vi "ObjDet_Read_Dataset.vi"(0 "Image Path(Train)":path, 1 "Validation Portion":sgl, 2 "Rndomize":bool=TRUE, 5 "Anno Path(Train)":path, 7 "Image Path(Test)":path, 9 "Anno Path(Test)":path, 11 "error in (no error)":errorcluster, 12 "Img Height":i32=128, 13 "Img Width":i32=128, 14 "Img Type":enum16{"Grayscale", "RGB"}(ring)) -> (4 "Dataset":T1={"Train"={"Inputs Ref."=variant(refnum<data-value> refnum), "Dataset_Size"=0, "Dims_In"={"C"=0, "H"=0, "W"=0}, "Outputs Refs"=refnum, "No of Classes "=0, "Labels"=["large", "small"], "File Paths"=[]}, "Validation"={"Inputs Ref."=variant(refnum<data-value> refnum), "Dataset_Size"=0, "Dims_In"={"C"=0, "H"=0, "W"=0}, "Outputs Refs"=refnum, "No of Classes "=0, "Labels"=["large", "small"], "File Paths"=[]}, "Test"={"Inputs Ref."=variant(refnum<data-value> refnum), "Dataset_Size"=0, "Dims_In"={"C"=0, "H"=0, "W"=0}, "Outputs Refs"=refnum, "No of Classes "=0, "Labels"=["large", "small"], "File Paths"=[]}}, 6 "Anchors":dbl[][](array[numeric]), 8 "Total annotations":i32, 15 "error out":errorcluster)   [LabVIEW 2020]
uses:
  <vilib>/Ngene/Deep Learning Toolkit/Toolkit/NN_Data/API/DataSet/DataSet_Types/NN_DataSets_All(In3D_OutBBox).ctl
  <vilib>/Ngene/Deep Learning Toolkit/Toolkit/NN_Data/API/DataSet/DataSet_Types/NN_DataSet(In3D_OutBBox).ctl
  <vilib>/Ngene/Deep Learning Toolkit/Toolkit/NN_Data/API/NN_Dims(C,H,W).ctl
  <vilib>/Ngene/Deep Learning Toolkit/Toolkit/NN_Data/Controls/DataRef_Types/1D/NN_Data_ref(1D_BBox).ctl
  <vilib>/Ngene/Deep Learning Toolkit/Toolkit/NN_Data/API/Data/Detection_Types/NN_Image_Annotations.ctl
  <vilib>/Ngene/Deep Learning Toolkit/Toolkit/NN_Data/API/Data/Detection_Types/NN_BBox_Annotation.ctl
  <vilib>/Ngene/Deep Learning Toolkit/Toolkit/NN_Data/API/Data/Detection_Types/NN_BBox.ctl
  <vilib>/Analysis/1siggen.llb/Riffle Array (I32).vi
  <vilib>/Ngene/Deep Learning Toolkit/Toolkit/Deep_Learning_Toolkit_by_Ngene.lvlib
  <vilib>/Analysis/NI_AALBase.lvlib
panel:
  in  "seed":i32=-1
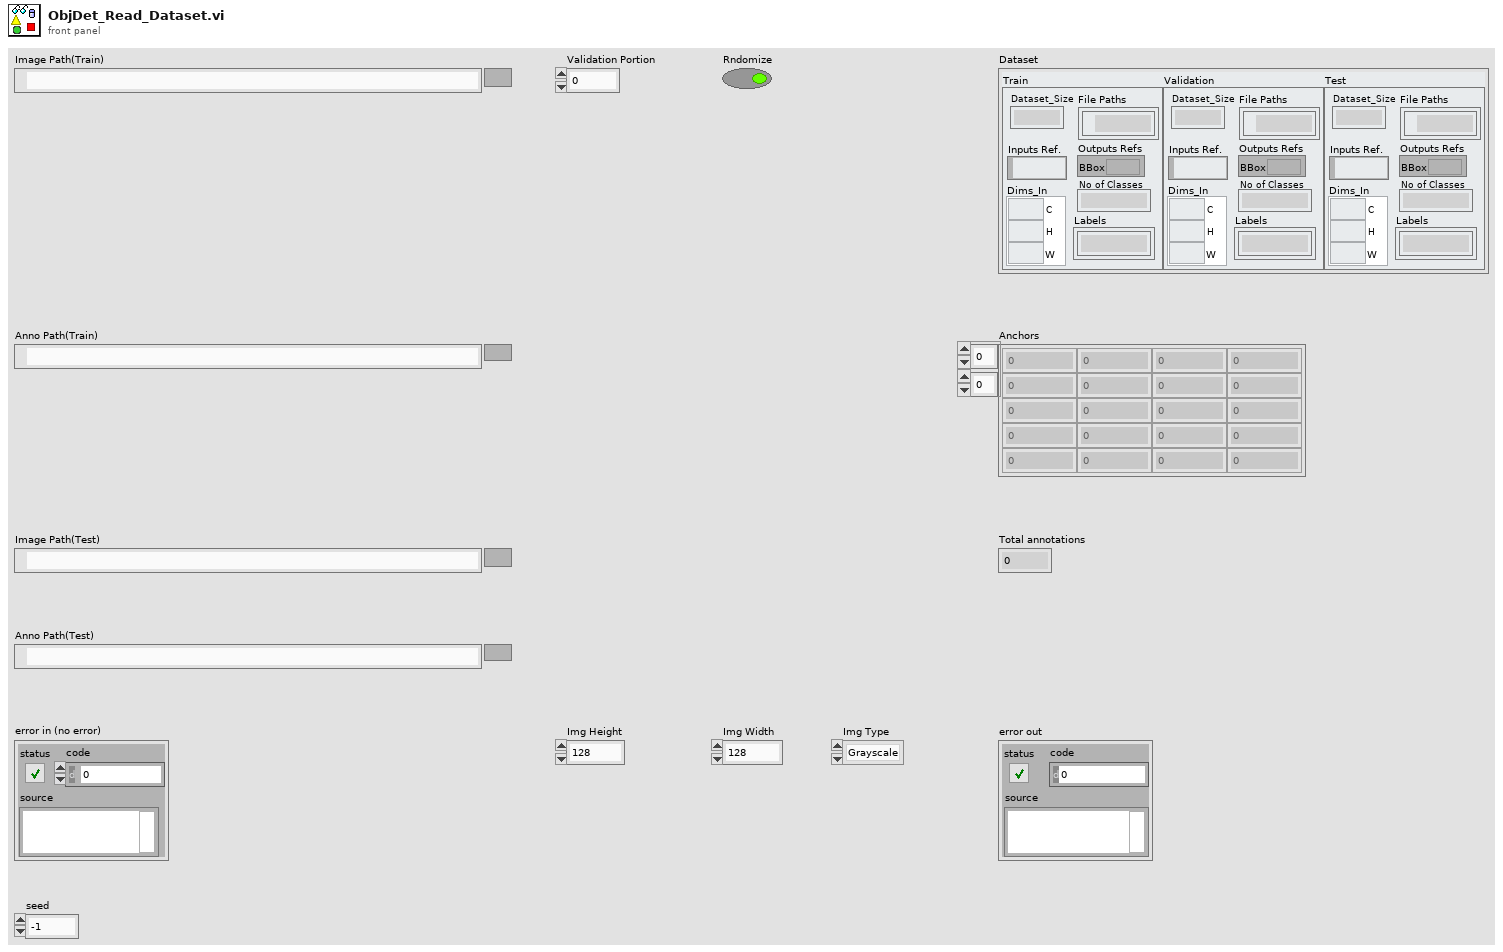
[diagram p1: front panel]
types:
  T1 = typedef "Deep_Learning_Toolkit_by_Ngene.lvlib/NN_DataSets_All(In3D_OutBBox).ctl" = cluster{"Train":T2, "Validation":T2, "Test":T2}
  T2 = typedef "Deep_Learning_Toolkit_by_Ngene.lvlib/NN_DataSet(In3D_OutBBox).ctl" = cluster{"Inputs Ref.":variant, "Dataset_Size":i32, "Dims_In":T3, "Outputs Refs":T4, "No of Classes ":i32, "Labels":string[], "File Paths":path[]}
  T3 = typedef "Deep_Learning_Toolkit_by_Ngene.lvlib/NN_Dims(C,H,W).ctl" = cluster{"C":i32, "H":i32, "W":i32}
  T4 = typedef "Deep_Learning_Toolkit_by_Ngene.lvlib/NN_Data_ref(1D_BBox).ctl" = refnum<data-value>
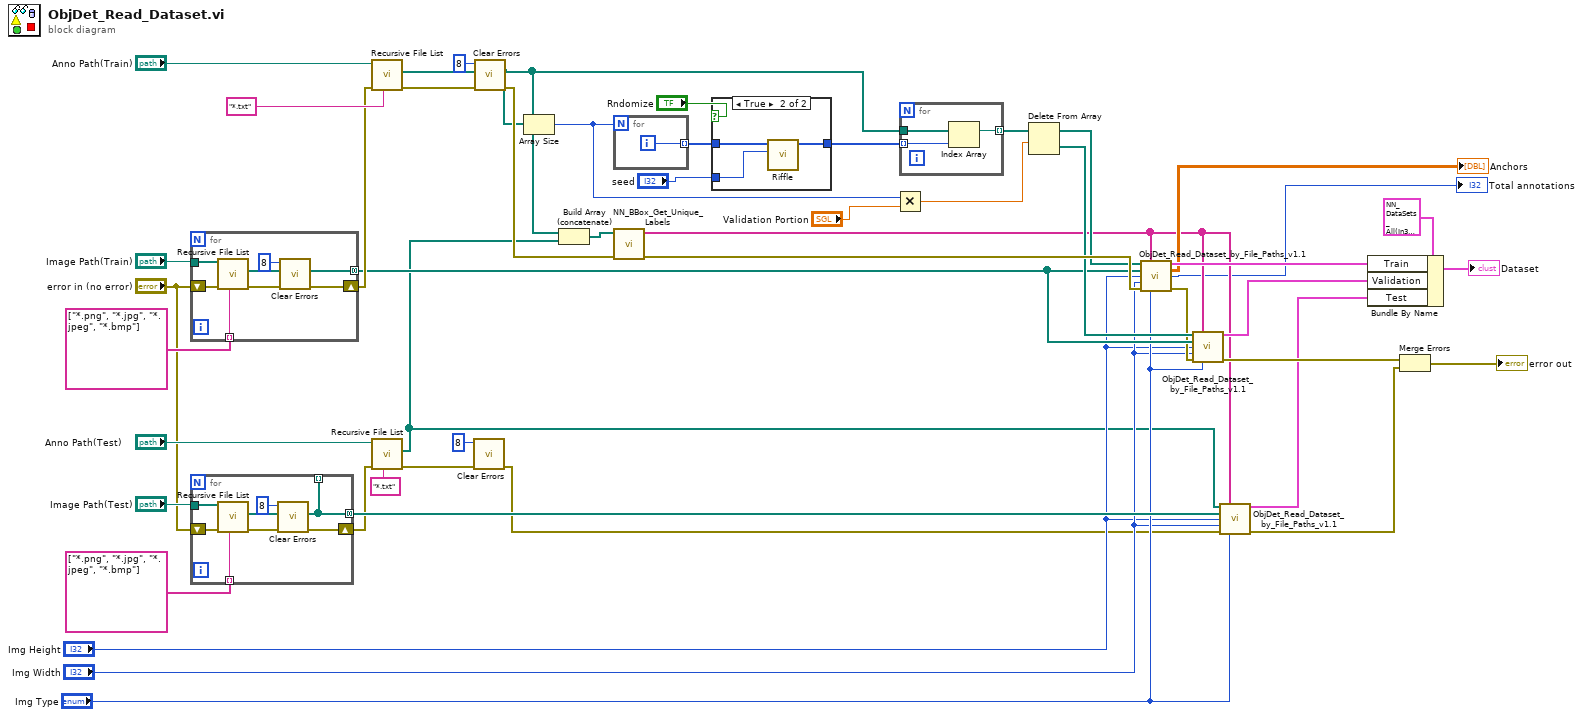
[diagram p0: block diagram]
diagram:
  n1 = for {
    tunnel: "Image Path(Train)" -> [w55]
    tunnel: string[] ["*.png", "*.jpg", "*.jpeg", "*.bmp"] ("pattern") -> [w54] mode=indexing
    tunnel: [w49] -> w31 mode=concatenating
    shift-right: [w51] -> w46
    shift-left: "error in (no error)" -> [w53]
    n2 = call <vilib>:"Recursive File List.vi"("pattern"=w54, "error in (no error)"=w53, "Folder Path"=w55) -> ("error out"=w52:errorcluster, "All Files in Dir"=w49:path[])  [unwired: 4 in, 3 out]
    n3 = call <vilib>:"Clear Errors.vi"("error in (no error)"=w52, "specific error code to clear (0: all)"=8) -> ("error out"=w51:errorcluster)  [unwired: 4 in, 1 out]
  }
  n4 = for {
    tunnel: "Image Path(Test)" -> [w62]
    tunnel: string[] ["*.png", "*.jpg", "*.jpeg", "*.bmp"] ("pattern") -> [w61] mode=indexing
    tunnel: [w56] -> w26 mode=concatenating
    shift-right: [w58] -> w23
    shift-left: "error in (no error)" -> [w60]
    tunnel: [w56] -> _ mode=indexing
    n5 = call <vilib>:"Recursive File List.vi"("pattern"=w61, "error in (no error)"=w60, "Folder Path"=w62) -> ("error out"=w59:errorcluster, "All Files in Dir"=w56:path[])  [unwired: 4 in, 3 out]
    n6 = call <vilib>:"Clear Errors.vi"("error in (no error)"=w59, "specific error code to clear (0: all)"=8) -> ("error out"=w58:errorcluster)  [unwired: 4 in, 1 out]
  }
  n7 = call <vilib>:"Recursive File List.vi"("pattern"="*.txt", "error in (no error)"=w46, "Folder Path"="Anno Path(Train)") -> ("error out"=w42:errorcluster, "All Files in Dir"=w3:path[])  [unwired: 4 in, 3 out]
  n8 = call <vilib>:"Recursive File List.vi"("pattern"="*.txt", "error in (no error)"=w23, "Folder Path"="Anno Path(Test)") -> ("error out"=w25:errorcluster, "All Files in Dir"=w1:path[])  [unwired: 4 in, 3 out]
  n9 = call <vilib>:"Clear Errors.vi"("error in (no error)"=w25, "specific error code to clear (0: all)"=8) -> ("error out"=w10:errorcluster)  [unwired: 4 in, 1 out]
  n10 = call <vilib>:"Clear Errors.vi"("error in (no error)"=w42, "specific error code to clear (0: all)"=8) -> ("error out"=w11:errorcluster)  [unwired: 4 in, 1 out]
  n11 = Array Size(array=w3) -> (size(s)=w38:i32)
  n12 = Build Array (concatenate)(w3, w1) -> (w2:path[])
  n13 = for {
    N: w38 -> [_]
    tunnel: [w63] -> w39 mode=indexing
    i -> [w63]
  }
  n14 = call "NN_BBox_Get_Unique_Labels.vi"("error in (no error)"=w11, "Anno File Paths"=w2) -> ("error out"=w41:errorcluster, "Unique labels"=w12:string[])  [unwired: 8 in]
  n15 = case shown="True" "Rndomize" {
    tunnel: w39 -> [w64 w67]
    tunnel: [w64 w66] -> w35
    tunnel: "seed" -> [_ w65]
    frame False {
    }
    frame True {
      n16 = call-poly <vilib>:"Riffle.vi"("seed"=w65, "X"=w67) -> ("Riffled {X}"=w66:i32[])  [unwired: 7 in, 2 out]
    }
  }
  n17 = Multiply(x=w38, y="Validation Portion") -> (x*y=w36:sgl)
  n18 = for {
    tunnel: [w69] -> w34 mode=indexing
    tunnel: w3 -> [w70]
    tunnel: w35 -> [w68] mode=indexing
    n19 = Index Array(array=w70, index=w68) -> (element=w69:path)
  }
  n20 = Delete From Array(array=w34, length=w36) -> (deleted portion=w32:path[], array with subset deleted=w33:path[])  [unwired: 1 in]
  n21 = call "ObjDet_Read_Dataset_by_File_Paths_v1.1.vi"("Annotation File Paths"=w33, "Unique labels"=w12, "Image File Paths"=w31, "Img Height"="Img Height", "Img Width"="Img Width", "error in (no error)"=w41, "Img Type"="Img Type") -> ("NN_DataSet(In3D_OutBBox)"=w40:T2, "Anchors"=→"Anchors":dbl[][], "Total annotations"=→"Total annotations":i32, "error out"=w30:errorcluster)  [unwired: 5 in]
  n22 = call "ObjDet_Read_Dataset_by_File_Paths_v1.1.vi"("Annotation File Paths"=w32, "Unique labels"=w12, "Image File Paths"=w31, "Img Height"="Img Height", "Img Width"="Img Width", "error in (no error)"=w30, "Img Type"="Img Type") -> ("NN_DataSet(In3D_OutBBox)"=w28:T2, "error out"=w29:errorcluster)  [unwired: 5 in, 2 out]
  n23 = call "ObjDet_Read_Dataset_by_File_Paths_v1.1.vi"("Annotation File Paths"=w1, "Unique labels"=w12, "Image File Paths"=w26, "Img Height"="Img Height", "Img Width"="Img Width", "error in (no error)"=w10, "Img Type"="Img Type") -> ("NN_DataSet(In3D_OutBBox)"=w16:T2, "error out"=w17:errorcluster)  [unwired: 5 in, 2 out]
  n24 = Bundle By Name(cluster=T1 {"Train"={"Inputs Ref."=variant(refnum<data-value> refnum), "Dataset_Size"=0, "Dims_In"={"C"=0, "H"=0, "W"=0}, "Outputs Refs"=refnum, "No of Classes "=0, "Labels"=["large", "small"], "File Paths"=[]}, "Validation"={"Inputs Ref."=variant(refnum<data-value> refnum), "Dataset_Size"=0, "Dims_In"={"C"=0, "H"=0, "W"=0}, "Outputs Refs"=refnum, "No of Classes "=0, "Labels"=["large", "small"], "File Paths"=[]}, "Test"={"Inputs Ref."=variant(refnum<data-value> refnum), "Dataset_Size"=0, "Dims_In"={"C"=0, "H"=0, "W"=0}, "Outputs Refs"=refnum, "No of Classes "=0, "Labels"=["large", "small"], "File Paths"=[]}} ("Dataset_Refs_All(In3D_OutBBox)"), "Train"=w40, "Validation"=w28, "Test"=w16) -> (→"Dataset":T1)
  n25 = Merge Errors(w29, w17) -> (→"error out":errorcluster)
